vi "Ref_MaskP.vi"(0 "Mask Ch 1":refnum<vi>, 1 "Mask Ch 2":refnum<vi>, 2 "Mask Ch 3":refnum<vi>, 3 "Mask Ch 4":refnum<vi>, 4 "Mask Ch 5":refnum<vi>, 5 "Mask Ch 6":refnum<vi>, 6 "Mask Ch 7":refnum<vi>, 7 "Mask Ch 8":refnum<vi>, 8 "Mask Ch 9":refnum<vi>, 9 "Mask Ch 10":refnum<vi>, 10 "Mask Ch 11":refnum<vi>, 11 "Mask Ch 12":refnum<vi>, 14 "Init_F":bool=TRUE) -> (16 "Mask Ch 11 out":refnum<vi>, 17 "Mask Ch 12 out":refnum<vi>, 18 "Mask Ch 9 out":refnum<vi>, 19 "Mask Ch 10 out":refnum<vi>, 20 "Mask Ch 1 out":refnum<vi>, 21 "Mask Ch 2 out":refnum<vi>, 22 "Mask Ch 3 out":refnum<vi>, 23 "Mask Ch 4 out":refnum<vi>, 24 "Mask Ch 5 out":refnum<vi>, 25 "Mask Ch 6 out":refnum<vi>, 26 "Mask Ch 7 out":refnum<vi>, 27 "Mask Ch 8 out":refnum<vi>)   [LabVIEW 2017]
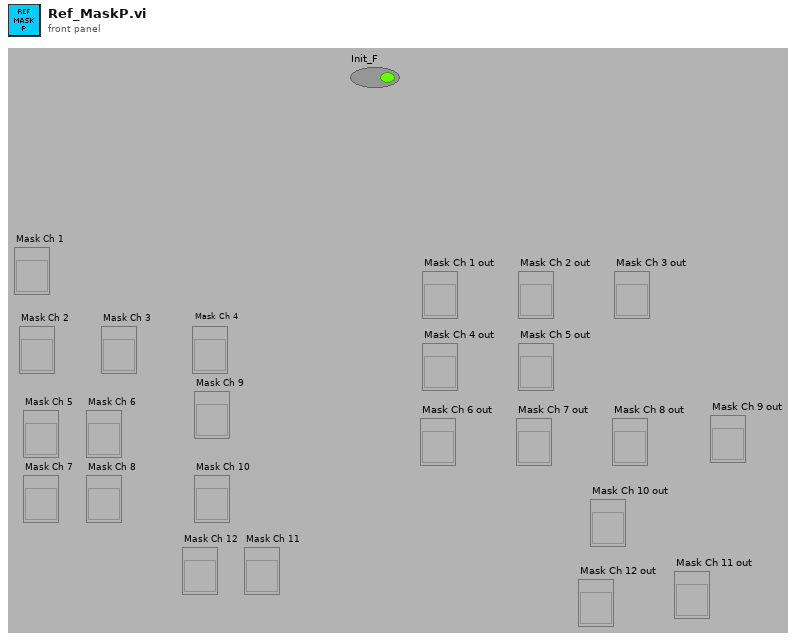
[diagram p1: front panel]
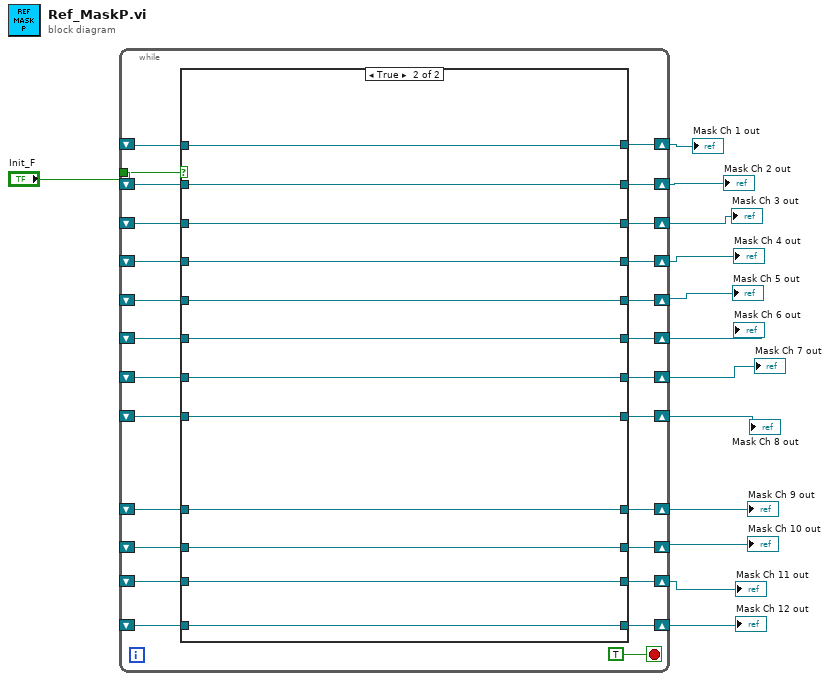
[diagram p0: block diagram]
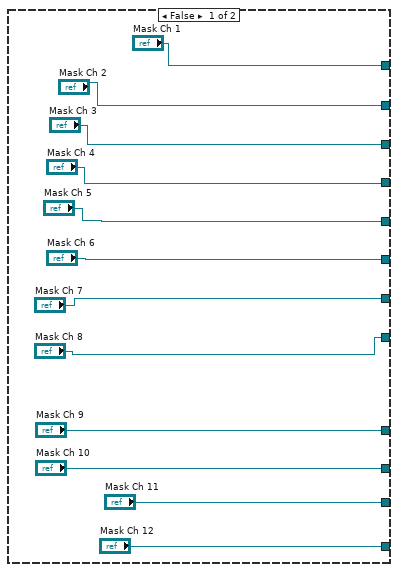
[diagram p2: hidden frame]
diagram:
  n1 = while {
    shift-right: [w38] -> w12
    shift-left: _ -> [w37]
    tunnel: "Init_F" -> [w36]
    shift-right: [w35] -> w11
    shift-left: _ -> [w28]
    shift-right: [w34] -> w10
    shift-left: _ -> [w27]
    shift-right: [w33] -> w9
    shift-left: _ -> [w22]
    shift-right: [w32] -> w8
    shift-left: _ -> [w26]
    shift-right: [w31] -> w7
    shift-left: _ -> [w25]
    shift-right: [w30] -> w6
    shift-left: _ -> [w24]
    shift-right: [w29] -> w5
    shift-left: _ -> [w23]
    shift-right: [w21] -> w4
    shift-left: _ -> [w19]
    shift-right: [w20] -> w3
    shift-left: _ -> [w18]
    shift-right: [w17] -> w2
    shift-left: _ -> [w15]
    shift-right: [w16] -> w1
    shift-left: _ -> [w14]
    stop <- TRUE stop-if-true
    n2 = case shown="True" w36 {
      tunnel: ["Mask Ch 1" w63] -> w38
      tunnel: w37 -> [_ w63]
      tunnel: ["Mask Ch 2" w56] -> w35
      tunnel: ["Mask Ch 3" w57] -> w34
      tunnel: ["Mask Ch 4" w58] -> w33
      tunnel: ["Mask Ch 5" w59] -> w32
      tunnel: ["Mask Ch 6" w60] -> w31
      tunnel: ["Mask Ch 7" w61] -> w30
      tunnel: ["Mask Ch 8" w62] -> w29
      tunnel: w28 -> [_ w56]
      tunnel: w27 -> [_ w57]
      tunnel: w26 -> [_ w59]
      tunnel: w25 -> [_ w60]
      tunnel: w24 -> [_ w61]
      tunnel: w23 -> [_ w62]
      tunnel: w22 -> [_ w58]
      tunnel: ["Mask Ch 9" w55] -> w21
      tunnel: ["Mask Ch 10" w54] -> w20
      tunnel: w19 -> [_ w55]
      tunnel: w18 -> [_ w54]
      tunnel: ["Mask Ch 11" w53] -> w17
      tunnel: ["Mask Ch 12" w52] -> w16
      tunnel: w15 -> [_ w53]
      tunnel: w14 -> [_ w52]
      frame False {
      }
      frame True {
      }
    }
  }
  "Mask Ch 1 out" <- w12
  "Mask Ch 2 out" <- w11
  "Mask Ch 3 out" <- w10
  "Mask Ch 4 out" <- w9
  "Mask Ch 5 out" <- w8
  "Mask Ch 6 out" <- w7
  "Mask Ch 7 out" <- w6
  "Mask Ch 8 out" <- w5
  "Mask Ch 9 out" <- w4
  "Mask Ch 10 out" <- w3
  "Mask Ch 11 out" <- w2
  "Mask Ch 12 out" <- w1
